vi "Correct_Pos_info_from Adam Chs.vi"() -> (0 "error out":errorcluster, 4 "Path":path)   [LabVIEW 2018]
panel:
  out "Array":path[](array[path])
  out "File Changed":bool
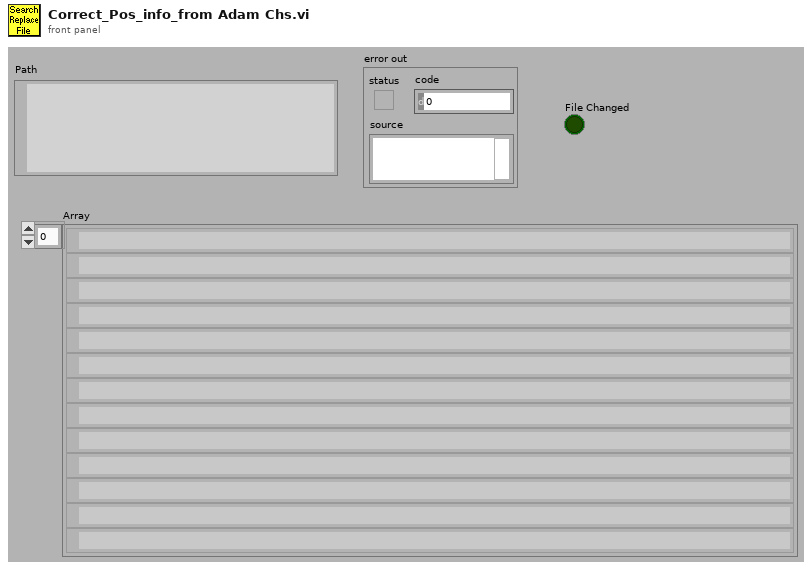
[diagram p1: front panel]
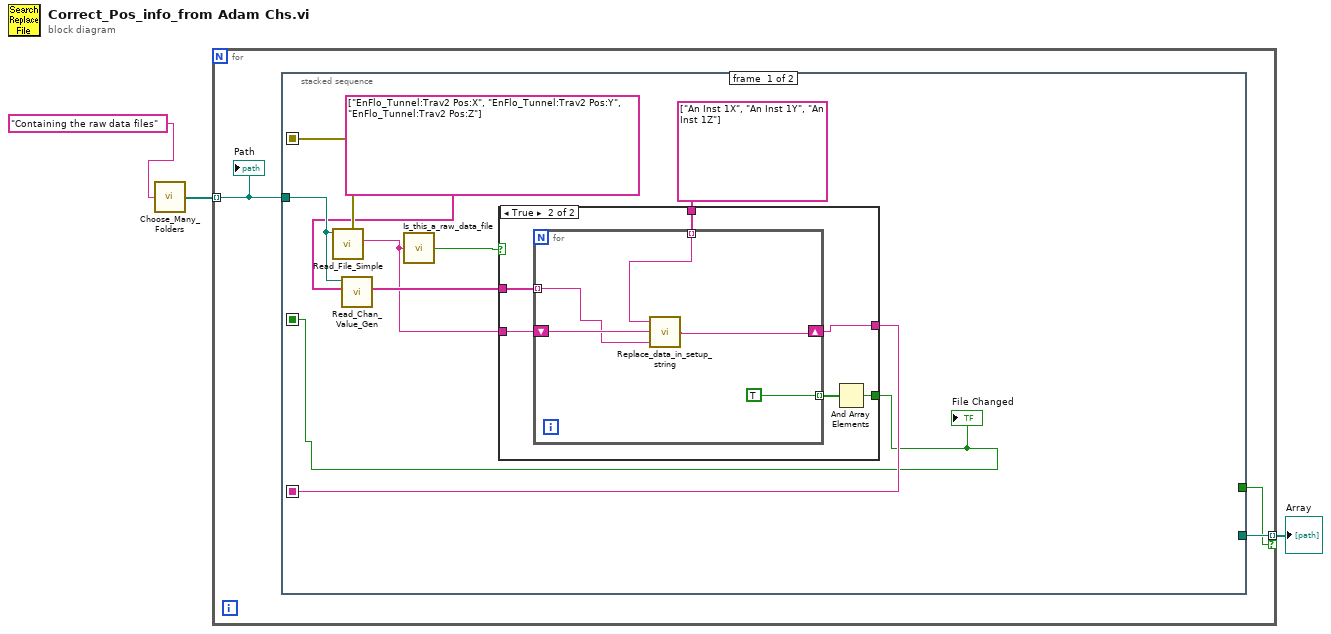
[diagram p0: block diagram]
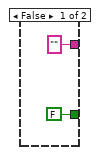
[diagram p2: hidden frame]
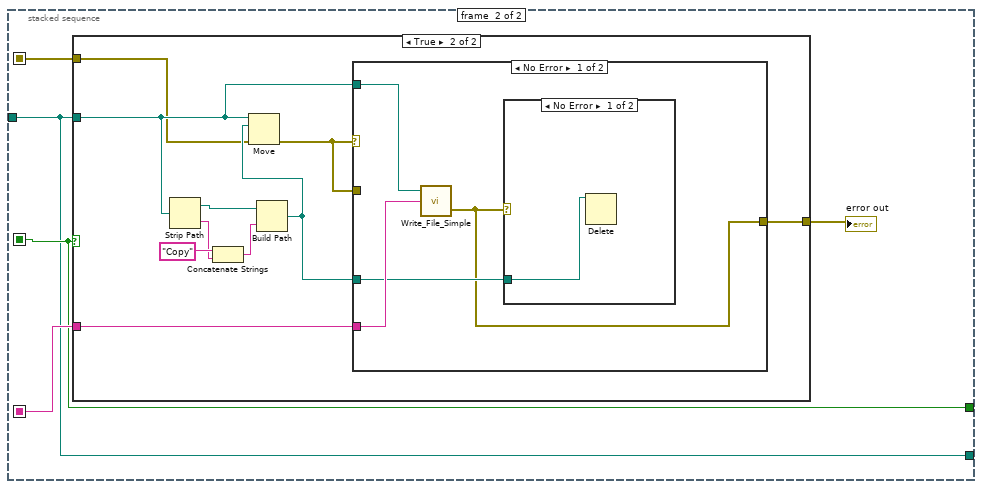
[diagram p3: hidden frame]
diagram:
  n1 = call "Choose_Many_Folders.vi"("Purpose of choosing folder"="Containing the raw data files") -> ("Files"=w2:path[])
  n2 = for {
    tunnel: w2 -> [w6] mode=indexing
    tunnel: [w5] -> w1 mode=indexing if=w4
    n3 = stacked-sequence {
      seq-local: [w15 _] -> [_ w32]
      seq-local: [w13 _] -> [_ w31]
      seq-local: [w12 _] -> [_ w30]
      tunnel: w6 -> [w11 w29]
      tunnel: [_ w29] -> w5
      tunnel: [_ w30] -> w4
      frame #0 {
        n4 = call "Read_File_Simple.vi"("Filename"=w11) -> ("error out"=w15:errorcluster, "string"=w8:string)  [unwired: 4 in, 4 out]
        n5 = call "Read_Chan_Value_Gen.vi"("Desired Ch Names"=string[] ["EnFlo_Tunnel:Trav2 Pos:X", "EnFlo_Tunnel:Trav2 Pos:Y", "EnFlo_Tunnel:Trav2 Pos:Z"], "Raw data file"=w11) -> ("Values"=w10:string[])  [unwired: 9 in]
        n6 = call "Is_this_a_raw_data_file.vi"("character string"=w8) -> ("Raw Dat File?"=w7:bool)  [unwired: 2 out]
        n7 = case shown="True" w7 {
          tunnel: string[] ["An Inst 1X", "An Inst 1Y", "An Inst 1Z"] -> [_ w23]
          tunnel: ["" ("string") w22] -> w13
          tunnel: [FALSE w20] -> w12
          tunnel: w10 -> [_ w19]
          tunnel: w8 -> [_ w18]
          frame False {
          }
          frame True {
            n8 = for {
              shift-right: [w24] -> w22
              shift-left: w18 -> [w27]
              tunnel: w23 -> [w28] mode=indexing
              tunnel: [TRUE] -> w21 mode=indexing
              tunnel: w19 -> [w25] mode=indexing
              n9 = call "Replace_data_in_setup_string.vi"("New data string"=w25, "Input string"=w27, "Variable name"=w28) -> ("Appended string"=w24:string)
            }
            n10 = And Array Elements(Boolean array=w21) -> (logical AND=w20:bool)
          }
        }
        "File Changed" <- w12
      }
      frame #1 {
        n11 = case shown="True" w30 {
          tunnel: w29 -> [_ w40]
          tunnel: w31 -> [_ w39]
          tunnel: [w34 w37] -> w33
          tunnel: w32 -> [w34 w35]
          frame False {
          }
          frame True {
            n12 = Strip Path(path=w40) -> (stripped path=w41:path, name=w43:string)
            n13 = Concatenate Strings("Copy" ("name or relative path"), w43) -> (w42:string)
            n14 = Build Path(base path=w41, name or relative path=w42) -> (appended path=w38:path)
            n15 = Move(source path=w40, error in=w35, 10:w38) -> (error out=w36:errorcluster)  [unwired: 2 in, 2 out]
            n16 = case shown="No Error" w36 {
              tunnel: w40 -> [w48 _]
              tunnel: w39 -> [w47 _]
              tunnel: w38 -> [w46 _]
              tunnel: [w45 w50] -> w37
              tunnel: w36 -> [_ w50]
              frame No Error {
                n17 = call "Write_File_Simple.vi"("character string"=w47, "file path"=w48) -> ("error out"=w45:errorcluster)  [unwired: 1 in, 1 out]
                n18 = case shown="No Error" w45 {
                  tunnel: w46 -> [w49 _]
                  frame No Error {
                    n19 = Delete(path (use dialog)=w49) -> ()  [unwired: 4 in, 3 out]
                  }
                  frame Error {
                  }
                }
              }
              frame Error {
              }
            }
          }
        }
        "error out" <- w33
      }
    }
    "Path" <- w6
  }
  "Array" <- w1
